vi "Go home.vi"(5 "Maximum wait time (45sec)":i32=45, 11 "error in (no error)":errorcluster) -> (15 "error out":errorcluster)   [LabVIEW 2024, in "GRBL 1.1.lvlib"]
doc: "Send go home command and report error if not done in the selected amount of time."
uses:
  GRBL 1.1.lvlib
panel:
  out "Data read":string
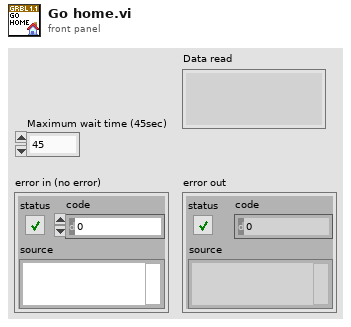
[diagram p1: front panel]
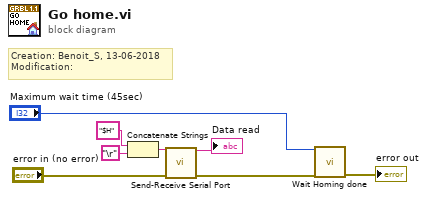
[diagram p0: block diagram]
diagram:
  # "Creation: Benoit_S, 13-06-2018\nModification:"
  n1 = Concatenate Strings("$H" ("Data to write"), "\r") -> (w6:string)
  n2 = call "Send-Receive Serial Port.vi"("Data to write"=w6, "error in (no error)"="error in (no error)") -> ("Data read"=→"Data read":string, "error out"=w1:errorcluster)  [unwired: 12 in]
  n3 = call "Wait Homing done.vi"("Maximum wait time (sec)"="Maximum wait time (45sec)", "error in (no error)"=w1) -> ("error out"=→"error out":errorcluster)  [unwired: 13 in]
